vi "dB Axis Scale.vi"(8 "Error In":errorcluster, 10 "Spectrum Scale\n[dB]":T1={-45.0, 50.0} scale=-80.0..20.0, 11 "Graph In":refnum<vi>) -> (0 "Error Out":errorcluster, 3 "Graph Out":refnum<vi>)   [LabVIEW 2017]
uses:
  Controls/dB Axis Scale.ctl
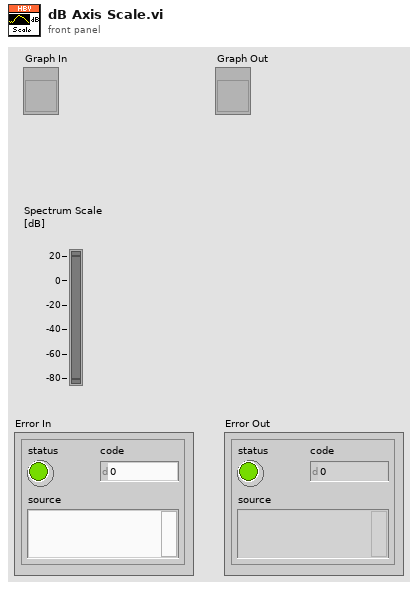
[diagram p1: front panel]
types:
  T1 = typedef "dB Axis Scale.ctl" = cluster{dbl, dbl}
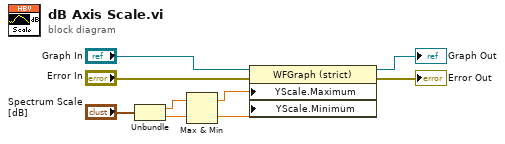
[diagram p0: block diagram]
diagram:
  n1 = Unbundle("Spectrum Scale\n[dB]") -> (w4:dbl, w5:dbl)
  n2 = Max & Min(x=w4, y=w5) -> (max(x,y)=w2:dbl, min(x,y)=w1:dbl)
  n3 = property on="Property Node" class="WFGraph (strict)"(reference="Graph In", error in="Error In", "YScale.Maximum"=w2, "YScale.Minimum"=w1) -> (reference out=→"Graph Out":refnum<vi>, error out=→"Error Out":errorcluster)
